vi "Write With Abort.vi"(6 "abort":bool, 10 "element":T1={"Temp. Sensirion"=0.01, "Hum. Sensirion"=0.01, "Temp. Switch Matrix"=0.01, "Hum. Switch Matrix"=0.01, "Temp. Probecard"=0.01, "Hum. Probecard"=0.01} {"Hum. Probecard" format="%#_13g"; "Temp. Probecard" format="%#_13g"; "Hum. Switch Matrix" format="%#_13g"; "Temp. Switch Matrix" format="%#_13g"; "Hum. Sensirion" format="%#_13g"; "Temp. Sensirion" format="%#_13g"}) -> (2 "channel":T2, 4 "aborted?":bool, 5 "previous element":T1={"Temp. Sensirion"=0.01, "Hum. Sensirion"=0.01, "Temp. Switch Matrix"=0.01, "Hum. Switch Matrix"=0.01, "Temp. Probecard"=0.01, "Hum. Probecard"=0.01} {"Hum. Probecard" format="%#_13g"; "Temp. Probecard" format="%#_13g"; "Hum. Switch Matrix" format="%#_13g"; "Temp. Switch Matrix" format="%#_13g"; "Hum. Sensirion" format="%#_13g"; "Temp. Sensirion" format="%#_13g"})   [LabVIEW 2020, in "Tag-t'data_env.ctl'.lvlib"]
doc: "Writes a value to a Tag channel or signals the channel to abort. This endpoint is the same as the Write endpoint except that it has an <B>abort</B> input and an <B>aborted?</B> output. You can use the abort capability of the Tag channel to close a channel abruptly, ignoring any data left in the channel buffer. You must use this endpoint together with the Read With Abort endpoint."
uses:
  <extravilib>/ChannelInstances/Tag-t'data_env.ctl'.lvlib
  <extravilib>/ChannelInstances/Tag-t'data_env.ctl'/))Channel.ctl
  Desktop/HexDAQ/src/data_env.ctl
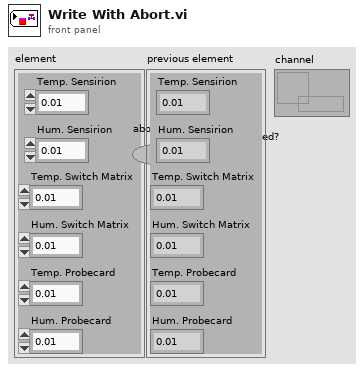
[diagram p1: front panel]
types:
  T1 = typedef "data_env.ctl" = cluster{"Temp. Sensirion":dbl, "Hum. Sensirion":dbl, "Temp. Switch Matrix":dbl, "Hum. Switch Matrix":dbl, "Temp. Probecard":dbl, "Hum. Probecard":dbl}
  T2 = typedef "Tag-t'data_env.ctl'.lvlib/))Channel.ctl" = refnum<queue>
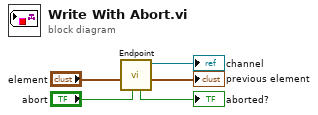
[diagram p0: block diagram]
diagram:
  n1 = call <extravilib>:"Endpoint.vi"("abort (F)"="abort", "element in"="element") -> ("element out"=→"previous element":T1, "channel out"=→"channel":T2, "aborted?"=→"aborted?":bool)  [unwired: 6 in, 1 out]
